vi "RSZVB Set TRM Pulse Modulator Source.vi"(7 "Pulse Modulator Source (Off)":i32(ring) items=["Off", "Internal Pulse Generator (via CASCADE IN)", "Internal Sync Generator (via CASCADE IN)", "External Generator 1 (via EXT PULSE GENERATOR 1)", "External Generator 2 (via EXT PULSE GENERATOR 2)"], 8 "error in (no error)":errorcluster {"code" format="%.0x"}, 9 "Path (1)":i32=1, 10 "Channel (1)":i32=1, 11 "VISA resource name":refnum<visa-resource-name>) -> (0 "error out":errorcluster {"code" format="%.0x"}, 3 "VISA resource name out":refnum<visa-resource-name>)   [LabVIEW 2011]
doc: "This VI selects the source (i.e. the pulse generator) for the pulse modulator at RF path <Path>.\n\nRemote-control command(s):\n[SENSe<Ch>:]TEUNit:PMODulator<Path>:SOURce"
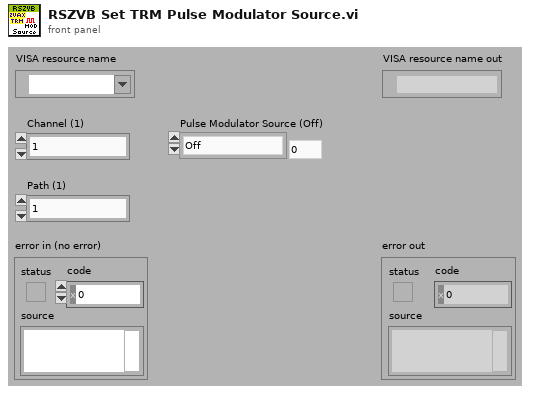
[diagram p1: front panel]
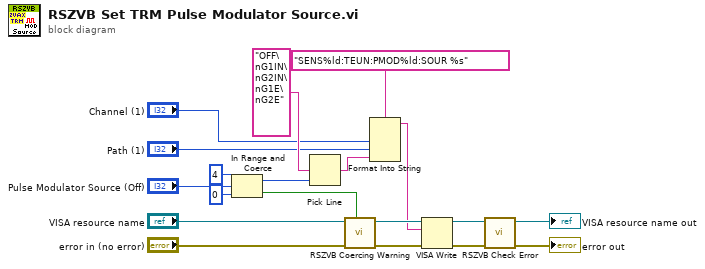
[diagram p0: block diagram]
diagram:
  n1 = In Range and Coerce(upper limit=4, x="Pulse Modulator Source (Off)", lower limit=0) -> (coerced(x)=w11:i32, In Range?=w15:bool)
  n2 = Pick Line(multi-line string="OFF\nG1IN\nG2IN\nG1E\nG2E", line index=w11) -> (output string=w10:string)  [unwired: 1 in]
  n3 = call "RSZVB Coercing Warning.vi"("In Range?"=w15, "error in (no error)"="error in (no error)", "VISA session"="VISA resource name") -> ("error out"=w18:errorcluster, "dup VISA session"=w19:refnum<visa-resource-name>)  [unwired: 7 in]
  n4 = Format Into String(format string="SENS%ld:TEUN:PMOD%ld:SOUR %s", "Channel (1)", "Path (1)", w10) -> (resulting string=w8:string)  [unwired: 2 in, 1 out]
  n5 = VISA Write(VISA resource name=w19, write buffer=w8, error in (no error)=w18) -> (VISA resource name out=w16:refnum<visa-resource-name>, error out=w17:errorcluster)  [unwired: 1 out]
  n6 = call "RSZVB Check Error.vi"("error in (no error)"=w17, "VISA session"=w16) -> ("error out"=→"error out":errorcluster, "dup VISA session"=→"VISA resource name out":refnum<visa-resource-name>)  [unwired: 8 in]
